vi "swerve_open_module.vi"(0 "Module Suffix":string, 5 "Drive CAN ID":u8, 7 "Azimuth CAN ID":u8, 9 "Encoder CAN ID":u8, 11 "error in":errorcluster, 12 "Encoder Offset (Deg)":dbl) -> (15 "error out":errorcluster)   [LabVIEW 2020]
uses:
  <vilib>/Rock Robotics/WPI/ThirdParty/Phoenix-LabVIEW/Motor Controller/Controls/CTRE_Phoenix_MotorControl_RemoteSourceType.ctl
  <vilib>/Rock Robotics/WPI/ThirdParty/Phoenix-LabVIEW/Motor Controller/Controls/CTRE_Phoenix_MotorControl_FeedbackDevice_TalonFX.ctl
  <vilib>/Rock Robotics/WPI/ThirdParty/Phoenix-LabVIEW/CANCoder/Controls/CTRE_Phoenix_CANcoder_SensorInitializationStrategy.ctl
  <vilib>/Rock Robotics/WPI/ThirdParty/Phoenix-LabVIEW/Motor Controller/Controls/CTRE_Phoenix_MotorControl_NeutralMode.ctl
  <vilib>/Rock Robotics/WPI/ThirdParty/Phoenix-LabVIEW/CANCoder/Controls/CTRE_Phoenix_CANcoder_StatusFrame.ctl
  <vilib>/Rock Robotics/WPI/ThirdParty/Phoenix-LabVIEW/Motor Controller/Controls/CTRE_Phoenix_MotorControl_StatusFrameEnhanced.ctl
  Status Frame Stuff/STATUS_Period.ctl
  Status Frame Stuff/Talon Status Frame Setting.ctl
  Status Frame Stuff/Talon Status Config Array.ctl
  <vilib>/Rock Robotics/WPI/ThirdParty/Phoenix-LabVIEW/CANCoder/Controls/CTRE_Phoenix_CANcoder_AbsoluteSensorRange.ctl
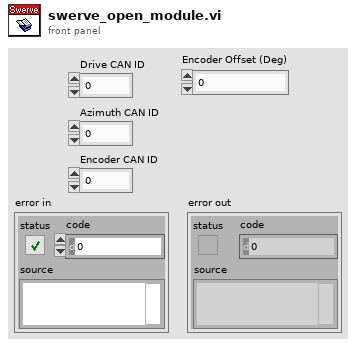
[diagram p1: front panel]
types:
  T1 = typedef "CTRE_Phoenix_CANcoder_AbsoluteSensorRange.ctl" = enum16{"Unsigned [0 to 360)", "Signed [-180 to +180)"}
  T2 = typedef "Talon Status Config Array.ctl" = T3[]
  T3 = typedef "Talon Status Frame Setting.ctl" = cluster{"Status Frame Enum":T4, "STATUS_Period":T5}
  T4 = typedef "CTRE_Phoenix_MotorControl_StatusFrameEnhanced.ctl" = u16
  T5 = typedef "STATUS_Period.ctl" = i32
  T6 = typedef "CTRE_Phoenix_CANcoder_StatusFrame.ctl" = u32
  T7 = typedef "CTRE_Phoenix_MotorControl_NeutralMode.ctl" = enum8{"EEPROMSetting", "Override to Coast", "Override to Brake"}
  T8 = typedef "CTRE_Phoenix_MotorControl_FeedbackDevice_TalonFX.ctl" = i8
  T9 = typedef "CTRE_Phoenix_MotorControl_RemoteSourceType.ctl" = enum16{"Off", "Talon SRX Selected Sensor", "Pigeon IMU Yaw", "Pigeon IMU Pitch", "Pigeon IMU Roll", "CANifier Quadrature", "CANifier PWM Input 0", "CANifier PWM Input 1", "CANifier PWM Input 2", "CANifier PWM Input 3", "Gadgeteer Pigeon Yaw", "Gadgeteer Pigeon Pitch", "Gadgeteer Pigeon Roll", "CANCoder"}
  T10 = typedef "CTRE_Phoenix_CANcoder_SensorInitializationStrategy.ctl" = enum16{"Boot To Zero", "Boot To Absolute Position"}
  T11 = typedef "WPI_MotorControlDeviceRef.ctl" = cluster{"DeviceStatus":errorcluster, "Type":T12, "PWM":cluster{"PWM Channel":T13, "DeadBand":T14}, "CAN":cluster{"Device Number":u8, "SetOutput VI Ref":variant, "GetOutput VI Ref":variant, "Enable VI Ref":variant, "Disable VI Ref":variant, "Data":variant}, "Invert":bool, "DIO PWM":cluster{"PWM \"Enable\" Channel":T13, "DIOChannel":T15, "PWM Rate":dbl}}
  T12 = typedef "WPI_MotorControlType.ctl" = enum16{"PWM", "CAN", "DIO PWM"}
  T13 = typedef "FPGA_DIOPWMChannel.ctl" = enum8{"PWM 0", "PWM 1", "PWM 2", "PWM 3", "PWM 4", "PWM 5", "PWM 6", "PWM 7", "PWM 8", "PWM 9", "PWM MXP 0", "PWM MXP 1", "PWM MXP 2", "PWM MXP 3", "PWM MXP 4", "PWM MXP 5", "PWM MXP 6", "PWM MXP 7", "PWM MXP 8", "PWM MXP 9", "Invalid"}
  T14 = typedef "WPI_PWMDeadband.ctl" = cluster{"Name":string, "maxPositivePwm":i32, "minPositivePwm":i32, "centerPwm":i32, "maxNegativePwm":i32, "minNegativePwm":i32, "angularRange":u16}
  T15 = typedef "FPGA_DIOChannel.ctl" = enum8{"DIO 0", "DIO 1", "DIO 2", "DIO 3", "DIO 4", "DIO 5", "DIO 6", "DIO 7", "DIO 8", "DIO 9", "DIO MXP 0", "DIO MXP 1", "DIO MXP 2", "DIO MXP 3", "DIO MXP 4", "DIO MXP 5", "DIO MXP 6", "DIO MXP 7", "DIO MXP 8", "DIO MXP 9", "DIO MXP 10", "DIO MXP 11", "DIO MXP 12", "DIO MXP 13", "DIO MXP 14", "DIO MXP 15", "SPI Port CS1", "SPI Port CS2", "SPI Port CS3", "SPI Port MISO", "SPI Port MOSI", "Invalid"}
  T16 = typedef "CTRE_Phoenix_CANcoder_DeviceRef.ctl" = cluster{"DeviceStatus":errorcluster, "Device Number":u8, "Handle":u64, "UsageFrame":u32, "Library Path":path}
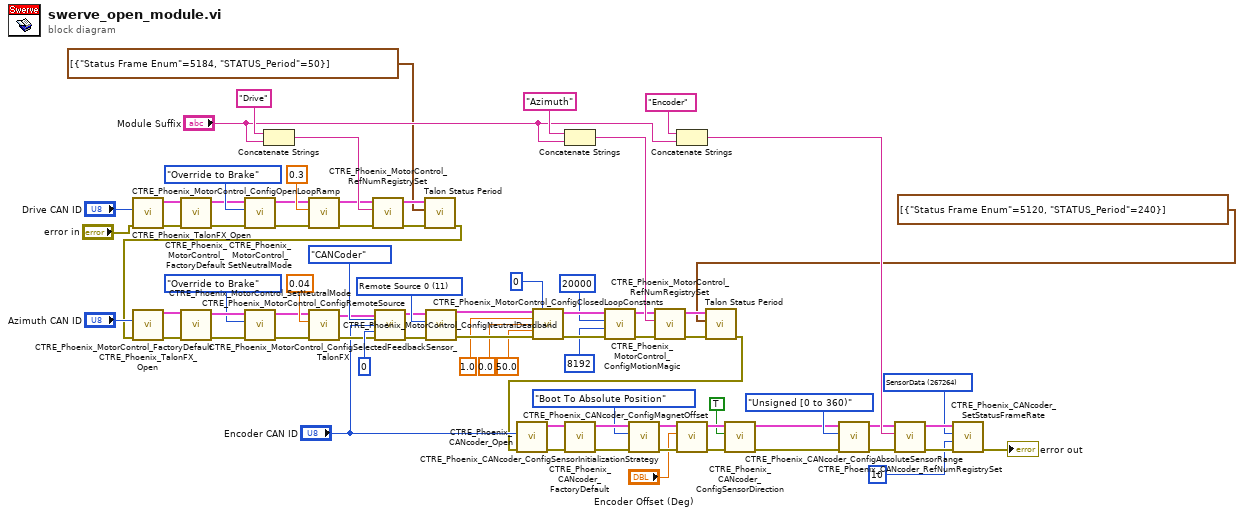
[diagram p0: block diagram]
diagram:
  w10 = T6 267264 items=["SensorData"=267264, "VbatAndFaults"=267328] ("CANcoder Status Frame")
  w54 = T8 11 items=["Integrated Sensor"=1, "Sensor Sum (S0 + S1)"=9, "Sensor Difference (D0 - D1)"=10, "Remote Source 0"=11, "Remote Source 1"=12, "None"=14, "Software Emulated"=15] ("Talon FX Feedback Device")
  n1 = call <vilib>:"CTRE_Phoenix_TalonFX_Open.vi"("error in"="error in", "Device Number"="Drive CAN ID") -> ("error out"=w72:errorcluster, "PhoenixMotorControlDevRef"=w73:T11)  [unwired: 8 in]
  n2 = call <vilib>:"CTRE_Phoenix_MotorControl_FactoryDefault.vi"("error in"=w72, "PhoenixMotorControlDevRef"=w73) -> ("error out"=w25:errorcluster, "PhoenixMotorControlDevRef"=w26:T11)  [unwired: 8 in]
  n3 = call <vilib>:"CTRE_Phoenix_MotorControl_SetNeutralMode.vi"("error in (no error)"=w25, "Motor Control Neutral Mode"=CTRE_Phoenix_MotorControl_NeutralMode."Override to Brake", "PhoenixMotorControlDevRef"=w26) -> ("error out"=w23:errorcluster, "PhoenixMotorControlDevRef"=w24:T11)  [unwired: 7 in]
  n4 = Concatenate Strings("Drive" ("string"), "Module Suffix") -> (w74:string)
  n5 = call <vilib>:"CTRE_Phoenix_MotorControl_ConfigOpenLoopRamp.vi"("error in (no error)"=w23, "secondsFromNeutralToFull"=0.3 ("Drive Ramp (Sec)"), "PhoenixMotorControlDevRef"=w24) -> ("error out"=w21:errorcluster, "PhoenixMotorControlDevRef"=w22:T11)  [unwired: 7 in]
  n6 = call <vilib>:"CTRE_Phoenix_MotorControl_RefNumRegistrySet.vi"("error in (no error)"=w21, "refnum name"=w74, "PhoenixMotorControlDevRef"=w22) -> ("error out"=w17:errorcluster, "PhoenixMotorControlDevRef"=w18:T11)  [unwired: 7 in]
  n7 = call "Talon Status Period.vi"("error in (no error)"=w17, "Status Config Array"=T2 [{"Status Frame Enum"=5184, "STATUS_Period"=50}] ("Drive Status Config"), "PhoenixMotorControlDevRef"=w18) -> ("error out"=w16:errorcluster)  [unwired: 7 in, 1 out]
  n8 = call <vilib>:"CTRE_Phoenix_TalonFX_Open.vi"("error in"=w16, "Device Number"="Azimuth CAN ID") -> ("error out"=w71:errorcluster, "PhoenixMotorControlDevRef"=w70:T11)  [unwired: 8 in]
  n9 = call <vilib>:"CTRE_Phoenix_MotorControl_FactoryDefault.vi"("error in"=w71, "PhoenixMotorControlDevRef"=w70) -> ("error out"=w44:errorcluster, "PhoenixMotorControlDevRef"=w45:T11)  [unwired: 8 in]
  n10 = call <vilib>:"CTRE_Phoenix_MotorControl_SetNeutralMode.vi"("error in (no error)"=w44, "Motor Control Neutral Mode"=CTRE_Phoenix_MotorControl_NeutralMode."Override to Brake", "PhoenixMotorControlDevRef"=w45) -> ("error out"=w42:errorcluster, "PhoenixMotorControlDevRef"=w43:T11)  [unwired: 7 in]
  n11 = call <vilib>:"CTRE_Phoenix_MotorControl_ConfigNeutralDeadband.vi"("error in (no error)"=w42, "Percent Deadband"=0.04, "PhoenixMotorControlDevRef"=w43) -> ("error out"=w39:errorcluster, "PhoenixMotorControlDevRef"=w40:T11)  [unwired: 7 in]
  n12 = call <vilib>:"CTRE_Phoenix_MotorControl_ConfigRemoteSource.vi"("PhoenixMotorControlDevRef"=w40, "Remote Device Type"=CTRE_Phoenix_MotorControl_RemoteSourceType."CANCoder", "Remote Device ID"="Encoder CAN ID", "Source Index (0/1)"=u32 0, "error in (no error)"=w39) -> ("PhoenixMotorControlDevRef"=w51:T11, "error out"=w50:errorcluster)  [unwired: 9 in]
  n13 = call <vilib>:"CTRE_Phoenix_MotorControl_ConfigSelectedFeedbackSensor_TalonFX.vi"("error in (no error)"=w50, "Talon FX Feedback Device"=w54, "PhoenixMotorControlDevRef"=w51) -> ("error out"=w37:errorcluster, "PhoenixMotorControlDevRef"=w38:T11)  [unwired: 7 in]
  n14 = call <vilib>:"CTRE_Phoenix_MotorControl_ConfigClosedLoopConstants.vi"("PhoenixMotorControlDevRef"=w38, "slotIdx"=0, "P"=1.0, "I"=0.0 ("P"), "D"=50.0 ("P"), "error in (no error)"=w37) -> ("PhoenixMotorControlDevRef"=w32:T11, "error out"=w31:errorcluster)  [unwired: 8 in]
  n15 = Concatenate Strings("Azimuth" ("string"), "Module Suffix") -> (w67:string)
  n16 = call <vilib>:"CTRE_Phoenix_MotorControl_ConfigMotionMagic.vi"("error in (no error)"=w31, "Acceleration"=8192 ("Cruise Velocity"), "Cruise Velocity"=20000, "PhoenixMotorControlDevRef"=w32) -> ("error out"=w27:errorcluster, "PhoenixMotorControlDevRef"=w28:T11)  [unwired: 6 in]
  n17 = call <vilib>:"CTRE_Phoenix_MotorControl_RefNumRegistrySet.vi"("error in (no error)"=w27, "refnum name"=w67, "PhoenixMotorControlDevRef"=w28) -> ("error out"=w14:errorcluster, "PhoenixMotorControlDevRef"=w15:T11)  [unwired: 7 in]
  n18 = Concatenate Strings("Encoder" ("string"), "Module Suffix") -> (w65:string)
  n19 = call "Talon Status Period.vi"("error in (no error)"=w14, "Status Config Array"=T2 [{"Status Frame Enum"=5120, "STATUS_Period"=240}] ("Drive Status Config"), "PhoenixMotorControlDevRef"=w15) -> ("error out"=w13:errorcluster)  [unwired: 7 in, 1 out]
  n20 = call <vilib>:"CTRE_Phoenix_CANcoder_Open.vi"("error in"=w13, "Device Number"="Encoder CAN ID") -> ("error out"=w47:errorcluster, "CTRE_CANcoder_DeviceRef"=w48:T16)  [unwired: 8 in]
  n21 = call <vilib>:"CTRE_Phoenix_CANcoder_FactoryDefault.vi"("error in"=w47, "CTRE_CANcoder_DeviceRef"=w48) -> ("error out"=w64:errorcluster, "CTRE_CANcoder_DeviceRef"=w63:T16)  [unwired: 8 in]
  n22 = call <vilib>:"CTRE_Phoenix_CANcoder_ConfigSensorInitializationStrategy.vi"("error in"=w64, "Sensor Initialization Strategy"=CTRE_Phoenix_CANcoder_SensorInitializationStrategy."Boot To Absolute Position", "CTRE_CANcoder_DeviceRef"=w63) -> ("error out"=w60:errorcluster, "CTRE_CANcoder_DeviceRef"=w59:T16)  [unwired: 7 in]
  n23 = call <vilib>:"CTRE_Phoenix_CANcoder_ConfigMagnetOffset.vi"("error in"=w60, "Magnet Offset (Degrees)"="Encoder Offset (Deg)", "CTRE_CANcoder_DeviceRef"=w59) -> ("error out"=w57:errorcluster, "CTRE_CANcoder_DeviceRef"=w56:T16)  [unwired: 7 in]
  n24 = call <vilib>:"CTRE_Phoenix_CANcoder_ConfigSensorDirection.vi"("error in"=w57, "Sensor Direction"=TRUE, "CTRE_CANcoder_DeviceRef"=w56) -> ("error out"=w1:errorcluster, "CTRE_CANcoder_DeviceRef"=w2:T16)  [unwired: 7 in]
  n25 = call <vilib>:"CTRE_Phoenix_CANcoder_ConfigAbsoluteSensorRange.vi"("error in"=w1, "Absolute Sensor Range"=CTRE_Phoenix_CANcoder_AbsoluteSensorRange."Unsigned [0 to 360)", "CTRE_CANcoder_DeviceRef"=w2) -> ("error out"=w5:errorcluster, "CTRE_CANcoder_DeviceRef"=w4:T16)  [unwired: 7 in]
  n26 = call <vilib>:"CTRE_Phoenix_CANcoder_RefNumRegistrySet.vi"("error in (no error)"=w5, "refnum name"=w65, "CTRE_CANcoder_DeviceRef"=w4) -> ("error out"=w12:errorcluster, "CTRE_CANcoder_DeviceRef"=w11:T16)  [unwired: 7 in]
  n27 = call <vilib>:"CTRE_Phoenix_CANcoder_SetStatusFrameRate.vi"("error in (no error)"=w12, "Period (ms)"=u8 10, "CANcoder Status Frame"=w10, "CTRE_CANcoder_DeviceRef"=w11) -> ("error out"=→"error out":errorcluster)  [unwired: 6 in, 1 out]
